vi "Create Symbolic Link.vi"(6 "timeout (ms)":i32=30000, 8 "error in":errorcluster, 9 "source":string, 10 "target":string, 11 "session in":refnum<class "Session.lvclass">) -> (0 "error out":errorcluster, 3 "session out":refnum<class "Session.lvclass">)   [LabVIEW 2020, in "NI_SFTP.lvlib"]
doc: "Creates a remote symbolic link."
uses:
  <vilib>/net/SFTP/NI_SFTP.lvlib
  <vilib>/net/SFTP/Session/Session.lvclass
  <vilib>/net/SFTP/API/Support/Command/SSH_FXP_SYMLINK/Input.ctl
  <vilib>/Utility/error.llb/Error Cluster From Error Code.vi
  <vilib>/ErrorRing/Error Ring.xnode
  <vilib>/net/SFTP/API/Support/Command/SSH_FXP_SYMLINK/SSH_FXP_SYMLINK.lvclass
  <vilib>/Utility/Deadline/NI_Deadline.lvlib
  <vilib>/net/SFTP/API/Support/Command/SSH_FXP_STAT/SSH_FXP_STAT.lvclass
  <vilib>/net/SSH/NI_SSH.lvlib
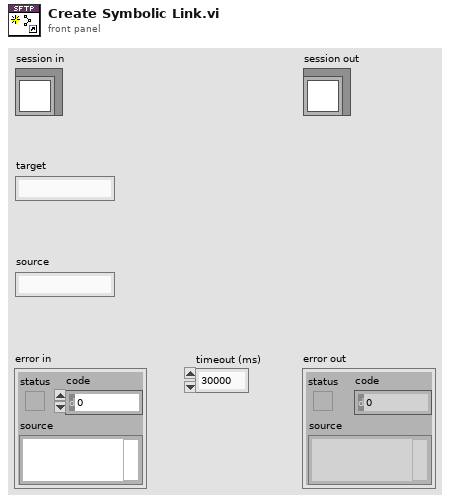
[diagram p1: front panel]
types:
  T1 = typedef "NI_SFTP.lvlib/SSH_FXP_SYMLINK.lvclass/Input.ctl" = cluster{"link path":string, "target path":string}
  T2 = typedef "NI_Deadline.lvlib/Deadline.ctl" = cluster{"mode":T3, "deadline (ms)":u32}
  T3 = typedef "NI_Deadline.lvlib/Mode.ctl" = enum16{"Relative", "Use deadline", "Wait forever", "Nonblocking", "N/A"}
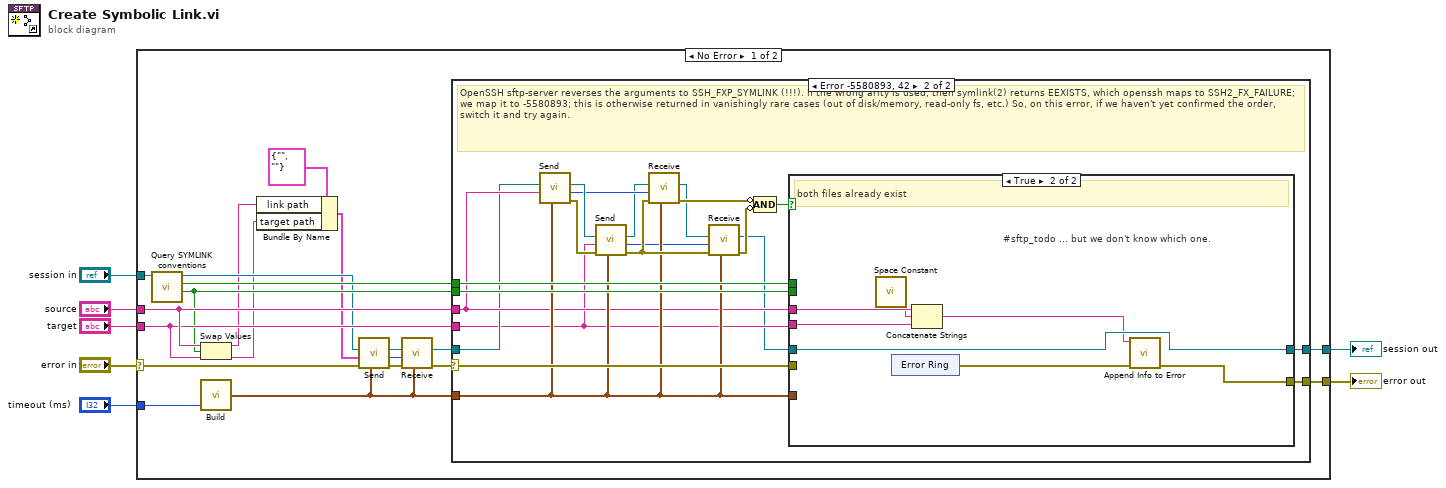
[diagram p0: block diagram]
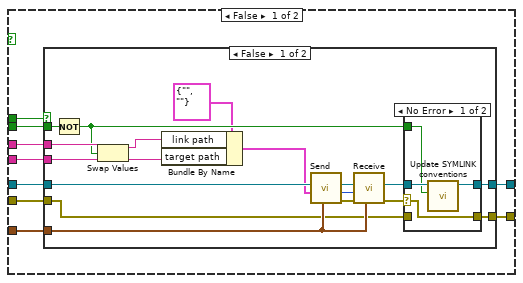
[diagram p3: hidden frame]
diagram:
  n1 = case shown="No Error" "error in" {
    selector: "error in" -> [w26 w97]
    tunnel: [w20 w97] -> w6
    tunnel: [w21 w96] -> w4
    tunnel: "session in" -> [w23 w96]
    tunnel: "timeout (ms)" -> [w25 _]
    tunnel: "target" -> [w16 _]
    tunnel: "source" -> [w18 _]
    frame No Error {
      n2 = call <vilib>:"Query SYMLINK conventions.vi"("session in"=w23) -> ("OpenSSH?"=w15:bool, "detected?"=w19:bool, "session out"=w14:refnum<class "Session.lvclass">)  [unwired: 8 in]
      n3 = Swap Values(12:w18, 13:w15, 14:w16) -> (1:w10:string, 3:w9:string)
      n4 = call <vilib>:"Build.vi"("timeout (ms)"=w25) -> ("Deadline out"=w17:T2)  [unwired: 2 in]
      n5 = Bundle By Name(cluster=T1 {"link path"="", "target path"=""} ("input"), "link path"=w10, "target path"=w9) -> (w8:T1)
      n6 = call <vilib>:"Send.vi"("Timeout"=w17, "error in (no error)"=w26, "input"=w8, "session in"=w14) -> ("error out"=w27:errorcluster, "request id"=w13:u32, "session out"=w24:refnum<class "Session.lvclass">)  [unwired: 4 in, 1 out]
      n7 = call <vilib>:"Receive.vi"("deadline"=w17, "error in (no error)"=w27, "request id"=w13, "session in"=w24) -> ("error out"=w22:errorcluster, "session out"=w12:refnum<class "Session.lvclass">)  [unwired: 4 in, 2 out]
      n8 = case shown="Error -5580893, 42" w22 {
        selector: w22 -> [w28 w45]
        tunnel: w12 -> [w29 w37]
        tunnel: [w29 w48] -> w21
        tunnel: [w28 w47] -> w20
        tunnel: w19 -> [_ w49]
        tunnel: w18 -> [_ w38]
        tunnel: w17 -> [_ w39]
        tunnel: w16 -> [_ w35]
        tunnel: w15 -> [_ w46]
        frame #0 {
        }
        frame #1 {
          # "OpenSSH sftp-server reverses the arguments to SSH_FXP_SYMLINK (!!!). If the wrong arity is used, then symlink(2) returns EEXISTS, which openssh maps to SSH2_FX_FAILURE; we map it to -5580893; this is otherwise returned in vanishingly rare cases (out of disk/memory, read-only fs, etc.) So, on this error, if we haven't yet confirmed the order, switch it and try again."
          n9 = call <vilib>:"Send.vi"("deadline"=w39, "path"=w38, "session in"=w37) -> ("error out"=w44:errorcluster, "request id"=w33:u32, "session out"=w36:refnum<class "Session.lvclass">)  [unwired: 5 in, 1 out]
          n10 = call <vilib>:"Send.vi"("deadline"=w39, "error in (no error)"=w44, "path"=w35, "session in"=w36) -> ("error out"=w43:errorcluster, "request id"=w34:u32, "session out"=w32:refnum<class "Session.lvclass">)  [unwired: 4 in, 1 out]
          n11 = call <vilib>:"Receive.vi"("deadline"=w39, "error in (no error)"=w43, "request id"=w33, "session in"=w32) -> ("error out"=w41:errorcluster, "session out"=w31:refnum<class "Session.lvclass">)  [unwired: 4 in, 2 out]
          n12 = call <vilib>:"Receive.vi"("deadline"=w39, "error in (no error)"=w43, "request id"=w34, "session in"=w31) -> ("error out"=w42:errorcluster, "session out"=w30:refnum<class "Session.lvclass">)  [unwired: 4 in, 2 out]
          n13 = Compound Arithmetic op=AND(invert w41, invert w42) -> (w40:bool)
          n14 = case shown="True" w40 {
            tunnel: w49 -> [w58 _]
            tunnel: [w57 w91] -> w48
            tunnel: [w56 w85] -> w47
            tunnel: w46 -> [w55 _]
            tunnel: w38 -> [w54 w90]
            tunnel: w45 -> [w53 _]
            tunnel: w39 -> [w52 _]
            tunnel: w30 -> [w51 w91]
            tunnel: w35 -> [w50 w89]
            frame False {
              n15 = case shown="False" w58 {
                tunnel: w51 -> [w65 w84]
                tunnel: w53 -> [w67 w83]
                tunnel: w52 -> [w74 _]
                tunnel: w54 -> [w73 _]
                tunnel: w50 -> [w72 _]
                tunnel: [w68 w84] -> w57
                tunnel: [w66 w83] -> w56
                tunnel: w55 -> [w71 _]
                frame False {
                  n16 = Not(x=w71) -> (.not. x?=w69:bool)
                  n17 = Swap Values(12:w73, 13:w69, 14:w72) -> (1:w63:string, 3:w62:string)
                  n18 = Bundle By Name(cluster=T1 {"link path"="", "target path"=""} ("input"), "link path"=w63, "target path"=w62) -> (w61:T1)
                  n19 = call <vilib>:"Send.vi"("Timeout"=w74, "input"=w61, "session in"=w65) -> ("error out"=w75:errorcluster, "request id"=w60:u32, "session out"=w76:refnum<class "Session.lvclass">)  [unwired: 5 in, 1 out]
                  n20 = call <vilib>:"Receive.vi"("deadline"=w74, "error in (no error)"=w75, "request id"=w60, "session in"=w76) -> ("error out"=w70:errorcluster, "session out"=w59:refnum<class "Session.lvclass">)  [unwired: 4 in, 2 out]
                  n21 = case shown="No Error" w70 {
                    selector: w70 -> [w77 _]
                    tunnel: w59 -> [w80 w82]
                    tunnel: w69 -> [w79 _]
                    tunnel: [w78 w82] -> w68
                    tunnel: w67 -> [_ w81]
                    tunnel: [w77 w81] -> w66
                    frame No Error {
                      n22 = call <vilib>:"Update SYMLINK conventions.vi"("OpenSSH detected"=w79, "session in"=w80) -> ("session out"=w78:refnum<class "Session.lvclass">)  [unwired: 9 in]
                    }
                    frame Error {
                    }
                  }
                }
                frame True {
                }
              }
            }
            frame True {
              # "#sftp_todo ... but we don't know which one."
              # "both files already exist"
              n23 = call <vilib>:"Space Constant.vi"() -> ("String"=w88:string)
              n24 = xnode "Error Ring"() -> ("error out"=w86:errorcluster)
              n25 = Concatenate Strings(w90, w88, w89) -> (w87:string)
              n26 = call <vilib>:"Append Info to Error.vi"("error in (no error)"=w86, "additional info"=w87) -> ("error out"=w85:errorcluster)  [unwired: 9 in]
            }
          }
        }
      }
    }
    frame Error {
    }
  }
  "error out" <- w6
  "session out" <- w4
